vi "Zaber Set-Go Home (SubVI).vi"(8 "error in (no error)":errorcluster, 10 "Set Home Offset":dbl, 11 "VISA Refnum in":refnum<visa-resource-name>) -> (0 "error out":errorcluster, 3 "VISA Refnum out":refnum<visa-resource-name>)   [LabVIEW 2012]
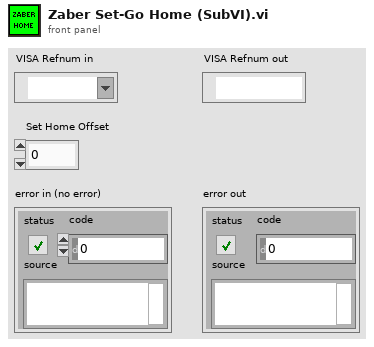
[diagram p1: front panel]
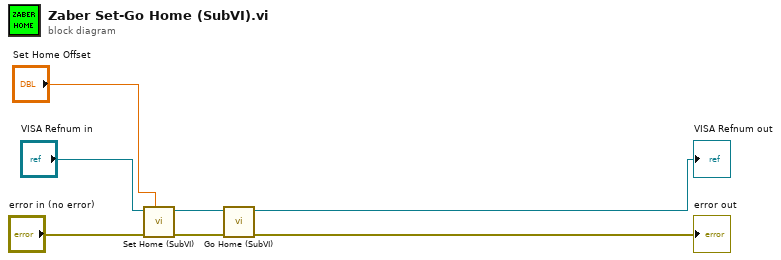
[diagram p0: block diagram]
diagram:
  n1 = call "Set Home (SubVI).vi"("Home Offset (deg)"="Set Home Offset", "error in (no error)"="error in (no error)", "VISA Refnum in"="VISA Refnum in") -> ("error out"=w2:errorcluster, "VISA Refnum out"=w3:refnum<visa-resource-name>)  [unwired: 7 in]
  n2 = call "Go Home (SubVI).vi"("error in (no error)"=w2, "VISA Refnum in"=w3) -> ("error out"=→"error out":errorcluster, "VISA Refnum out"=→"VISA Refnum out":refnum<visa-resource-name>)  [unwired: 8 in]
